vi "Serial Number Entry.vi"(8 "error in (no error)":errorcluster) -> (0 "error out":errorcluster, 2 "ok?":bool, 3 "Message In":string)   [LabVIEW 2021, in "User Interface.lvlib"]
uses:
  User Interface.lvlib
panel:
  in  "OK Button":bool
  in  "Cancel Button":bool
  in  "Serial Number":string
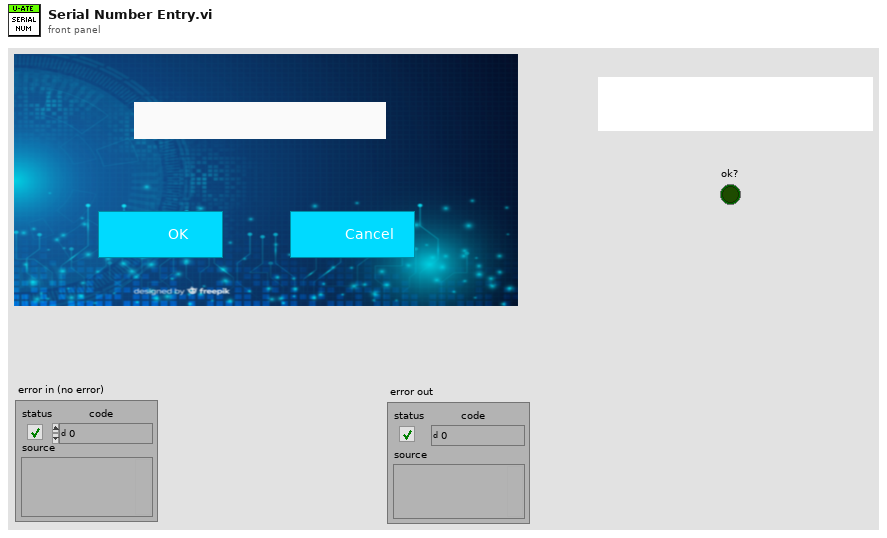
[diagram p1: front panel]
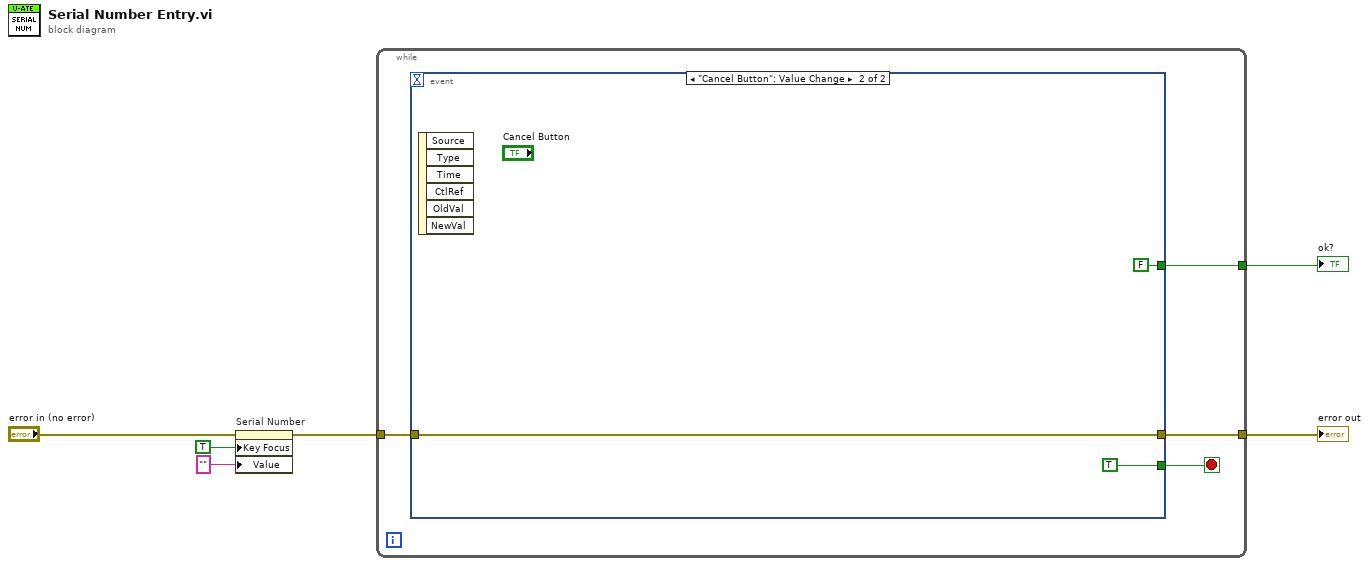
[diagram p0: block diagram]
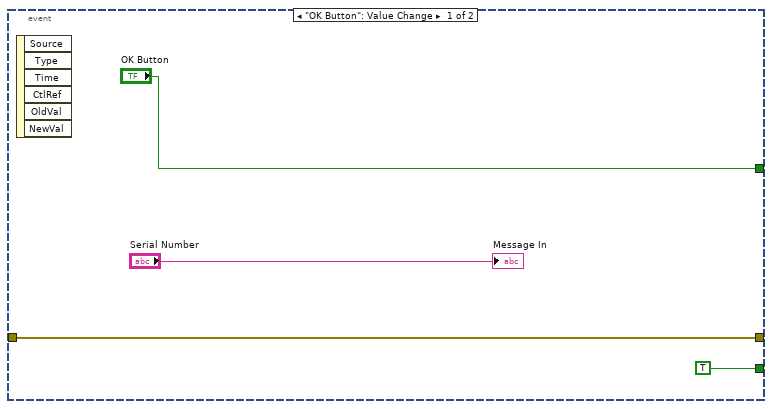
[diagram p2: hidden frame]
diagram:
  n1 = property on="Serial Number" class="Str"(error in="error in (no error)", "Key Focus"=TRUE, "Value"="" ("Serial Number")) -> (error out=w5:errorcluster)  [unwired: 1 in, 1 out]
  n2 = while {
    tunnel: w5 -> [w9]
    tunnel: [w8] -> w3
    tunnel: [w7] -> w2
    stop <- w10 stop-if-true
    n3 = event shown="[1] \"Cancel Button\": Value Change" {
      selector: _ -> [_ _]
      dyn-events: _ -> [_ _]
      timeout: _ -> [_ _]
      tunnel: [TRUE TRUE] -> w10
      tunnel: w9 -> [w12 w16]
      tunnel: [w12 w16] -> w8
      tunnel: ["OK Button" FALSE ("OK Button")] -> w7
      event "OK Button": Value Change {
        n4 = event-data() -> ()  [unwired: 1 in, 6 out]
        "Message In" <- "Serial Number"
      }
      event "Cancel Button": Value Change {
        n5 = event-data() -> ()  [unwired: 1 in, 6 out]
      }
    }
  }
  "error out" <- w3
  "ok?" <- w2
